vi "Add Event.vi"(5 "Log?":bool, 6 "Name":string, 7 "Value":string, 8 "Error In":errorcluster, 10 "Description":string, 11 "Boolean":bool) -> (0 "Error Out":errorcluster)   [LabVIEW 2019, in "GUI.lvlib"]
uses:
  GUI.lvlib
  Controls/Event.ctl
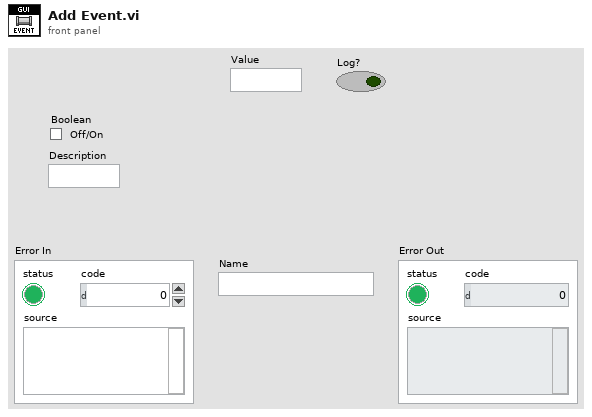
[diagram p1: front panel]
types:
  T1 = typedef "GUI.lvlib/Event.ctl" = cluster{"Name":string, "Time Stamp":timestamp, "Code":i32, "Source":string, "Value":string, "Boolean":bool, "Description":string, "Error":bool, "Warning":bool, " Fault":bool}
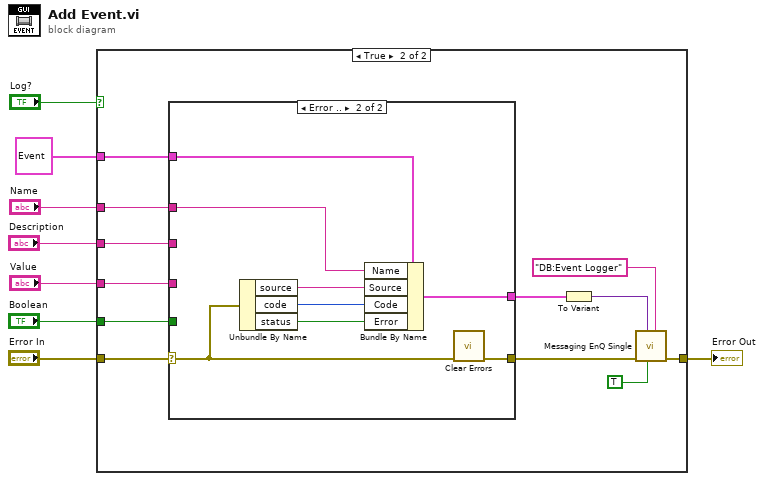
[diagram p0: block diagram]
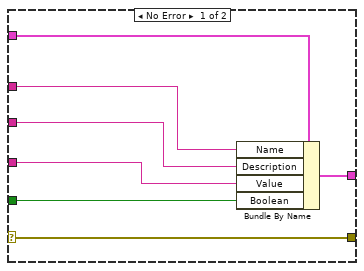
[diagram p3: hidden frame]
diagram:
  n1 = case shown="True" "Log?" {
    tunnel: "Error In" -> [w9 w21]
    tunnel: "Boolean" -> [_ w20]
    tunnel: "Value" -> [_ w19]
    tunnel: "Description" -> [_ w18]
    tunnel: "Name" -> [_ w17]
    tunnel: [w9 w15] -> w3
    tunnel: T1 {"Name"="", "Time Stamp"=timestamp(0 s since 1904-01-01), "Code"=0, "Source"="", "Value"="", "Boolean"=FALSE, "Description"="", "Error"=FALSE, "Warning"=FALSE, " Fault"=FALSE} ("Event") -> [_ w16]
    frame False {
    }
    frame True {
      n2 = case shown="Error .." w21 {
        selector: w21 -> [w23 w36]
        tunnel: [w23 w29] -> w14
        tunnel: w20 -> [w28 _]
        tunnel: w19 -> [w27 _]
        tunnel: w18 -> [w26 _]
        tunnel: w17 -> [w25 w32]
        tunnel: [w24 w31] -> w11
        tunnel: w16 -> [w22 w30]
        frame No Error {
          n3 = Bundle By Name(cluster=w22, "Name"=w25, "Description"=w26, "Value"=w27, "Boolean"=w28) -> (w24:T1)
        }
        frame Error {
          n4 = Unbundle By Name(w36) -> ("source"=w34:string, "code"=w35:i32, "status"=w33:bool)
          n5 = Bundle By Name(cluster=w30, "Name"=w32, "Source"=w34, "Code"=w35, "Error"=w33) -> (w31:T1)
          n6 = call <vilib>:"Clear Errors.vi"("error in (no error)"=w36) -> ("error out"=w29:errorcluster)  [unwired: 5 in, 1 out]
        }
      }
      n7 = To Variant(anything=w11) -> (Variant=w10:variant)
      n8 = call "Messaging EnQ Single.vi"("Command"="DB:Event Logger", "@Front?"=TRUE, "Data"=w10, "error in (no error)"=w14) -> ("error out"=w15:errorcluster)  [unwired: 7 in]
    }
  }
  "Error Out" <- w3
